vi "Convert Temperatures.vi"() -> ()   [LabVIEW 2012]
panel:
  out "Temperatures (Kelvin)":dbl[](array[numeric])
  in  "Temperatures (Celsius)":dbl[](array[numeric])=[-120.0, -200.0, -75.0, -45.0]
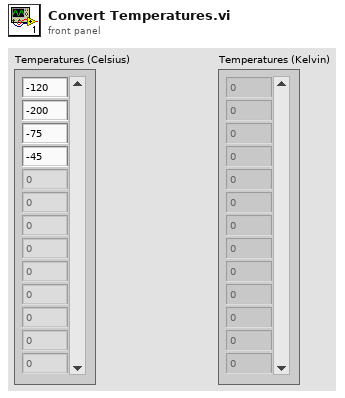
[diagram p1: front panel]
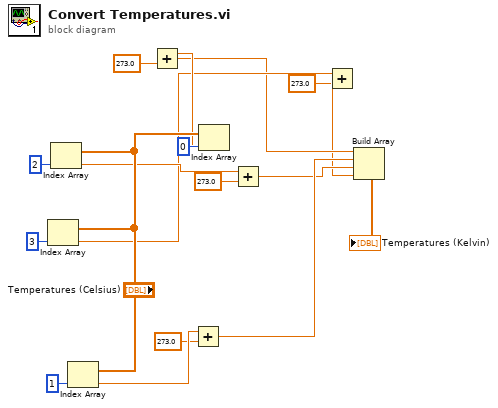
[diagram p0: block diagram]
diagram:
  n1 = Index Array(array="Temperatures (Celsius)", index=3) -> (element=w10:dbl)
  n2 = Index Array(array="Temperatures (Celsius)", index=2) -> (element=w11:dbl)
  n3 = Index Array(array="Temperatures (Celsius)", index=1) -> (element=w12:dbl)
  n4 = Add(x=w12, y=273.0) -> (x+y=w8:dbl)
  n5 = Index Array(array="Temperatures (Celsius)", index=0) -> (element=w13:dbl)
  n6 = Add(x=w13, y=273.0) -> (x+y=w9:dbl)
  n7 = Add(x=w11, y=273.0) -> (x+y=w7:dbl)
  n8 = Add(x=w10, y=273.0) -> (x+y=w6:dbl)
  n9 = Build Array(w9, w8, w7, w6) -> (→"Temperatures (Kelvin)":dbl[])
